vi "Conn Execute.vi"(5 "cache size (1)":i32=1 min=1, 6 "error in (no error)":errorcluster, 7 "cursor type":T3, 8 "SQL query":string, 9 "connection reference":T2) -> (0 "error out":errorcluster, 3 "recordset reference":T4)   [LabVIEW 2020, in "NI_Database_API.lvlib"]
doc: "Executes an SQL query and returns a recordset reference that you must eventually free with the DB Tools Free Object VI. Wire data to the reference input to determine the polymorphic instance to use or manually select the instance."
uses:
  <vilib>/addons/database/NI_Database_API.lvlib
  <vilib>/addons/database/Recordset.llb/Rec ObjectReference.ctl
  <vilib>/addons/database/Connection.llb/Conn ObjectReference.ctl
  <vilib>/addons/database/Auxilliary.llb/DB Tools Cursor Type.ctl
  <vilib>/addons/database/Recordset.llb/Rec DataMembers.ctl
panel:
  in  "default":T1
  in  "default data":T1
  in  "ADODB._Recordset":refnum<k7>
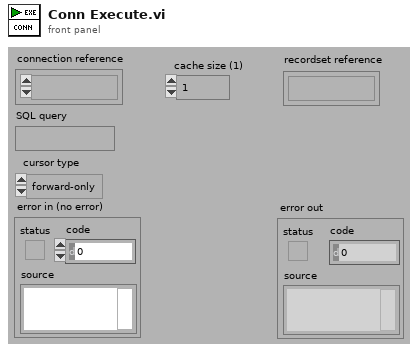
[diagram p1: front panel]
types:
  T1 = typedef "NI_Database_API.lvlib/Rec DataMembers.ctl" = cluster{"ADODB._Recordset":refnum<k7>, "Connection":T2}
  T2 = typedef "NI_Database_API.lvlib/Conn ObjectReference.ctl" = refnum<k1>
  T3 = typedef "NI_Database_API.lvlib/DB Tools Cursor Type.ctl" = enum16{"forward-only", "keyset", "dynamic", "static"}
  T4 = typedef "NI_Database_API.lvlib/Rec ObjectReference.ctl" = refnum<k1>
  T5 = typedef "NI_Database_API.lvlib/Conn DataMembers.ctl" = cluster{"ADODB._Connection":refnum<k7>, "recordset objects":i32, "command objects":i32}
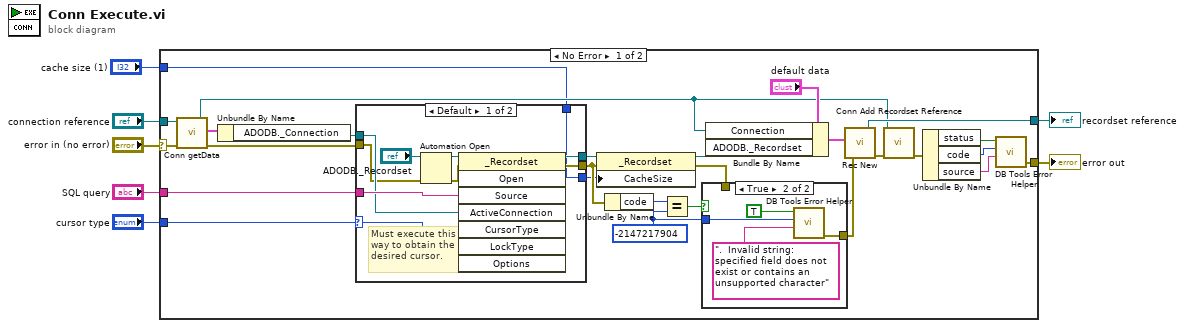
[diagram p0: block diagram]
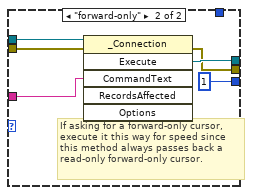
[diagram p3: hidden frame]
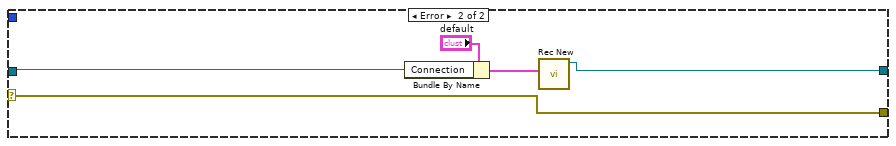
[diagram p4: hidden frame]
diagram:
  n1 = case shown="No Error" "error in (no error)" {
    selector: "error in (no error)" -> [w10 w60]
    tunnel: "cache size (1)" -> [w9 _]
    tunnel: [w32 w56] -> w1
    tunnel: "SQL query" -> [w30 _]
    tunnel: "cursor type" -> [w29 _]
    tunnel: "connection reference" -> [w26 w57]
    tunnel: [w12 w60] -> w3
    frame No Error {
      w19 = -2147217904
      n2 = call <vilib>:"Conn getData.vi"("error in (no error)"=w10, "connection reference"=w26) -> ("error out"=w25:errorcluster, "data"=w27:T5, "connection reference out"=w23:T2)  [unwired: 3 out]
      n3 = Unbundle By Name(w27) -> ("ADODB._Connection"=w24:refnum<k7>)
      n4 = case shown="Default" w29 {
        selector: w29 -> [w45 _]
        tunnel: w25 -> [w41 w54]
        tunnel: [w49 w53] -> w28
        tunnel: [w48 w52] -> w17
        tunnel: w30 -> [w47 w51]
        tunnel: w24 -> [w46 w55]
        tunnel: [w40 1 ("cache size (1)")] -> w8
        tunnel: w9 -> [w40 _]
        frame Default {
          # "Must execute this \nway to obtain the \ndesired cursor."
          n5 = Automation Open(error in (no error)=w41, Automation Refnum="ADODB._Recordset") -> (Automation Refnum=w43:refnum<k7>, error out=w42:errorcluster)  [unwired: 2 out]
          n6 = invoke class="_Recordset" method="Open"(reference=w43, error in=w42, "Source"=w47, "ActiveConnection"=w46, "CursorType"=w45) -> (reference out=w49:refnum<k7>, error out=w48:errorcluster)  [unwired: 3 in, 6 out]
        }
        frame "forward-only" {
          # "If asking for a forward-only cursor, \nexecute it this way for speed since \nthis method always passes back a \nread-only forward-only cursor."
          n7 = invoke class="_Connection" method="Execute"(reference=w55, error in=w54, "CommandText"=w51) -> (error out=w52:errorcluster, "Execute"=w53:refnum<k7>)  [unwired: 3 in, 4 out]
        }
      }
      n8 = property class="_Recordset"(reference=w28, error in=w17, "CacheSize"=w8) -> (reference out=w34:refnum<k7>, error out=w22:errorcluster)
      n9 = Unbundle By Name(w17) -> ("code"=w20:i32)
      n10 = Equal?(x=w20, y=w19) -> (x = y?=w18:bool)
      n11 = case shown="True" w18 {
        tunnel: w22 -> [w35 _]
        tunnel: [w35 w39] -> w21
        tunnel: w19 -> [_ w37]
        frame False {
        }
        frame True {
          n12 = call <vilib>:"DB Tools Error Helper.vi"("source"=".  Invalid string: specified field does not exist or contains an unsupported character", "code"=w37, "status"=TRUE) -> ("error out"=w39:errorcluster)  [unwired: 1 in, 7 out]
        }
      }
      n13 = Bundle By Name(cluster="default data", "Connection"=w23, "ADODB._Recordset"=w34) -> (w11:T1)
      n14 = call <vilib>:"Rec New.vi"("error in (no error)"=w21, "initial data"=w11) -> ("error out"=w33:errorcluster, "recordset reference"=w32:T4)  [unwired: 4 out]
      n15 = call <vilib>:"Conn Add Recordset Reference.vi"("error in (no error)"=w33, "connection reference"=w23) -> ("error out"=w13:errorcluster)  [unwired: 9 out]
      n16 = Unbundle By Name(w13) -> ("status"=w15:bool, "code"=w14:i32, "source"=w16:string)
      n17 = call <vilib>:"DB Tools Error Helper.vi"("source"=w16, "code"=w14, "status"=w15) -> ("error out"=w12:errorcluster)  [unwired: 1 in, 7 out]
    }
    frame Error {
      n18 = Bundle By Name(cluster="default", "Connection"=w57) -> (w59:T1)
      n19 = call <vilib>:"Rec New.vi"("initial data"=w59) -> ("recordset reference"=w56:T4)  [unwired: 1 in, 5 out]
    }
  }
  "recordset reference" <- w1
  "error out" <- w3
